vi "Initialisation Spectro.vi"(8 "error in (no error)":errorcluster caption="entrée d'erreur (pas d'erreur)", 10 "Connecter?":bool, 11 "UI SA en entrée":refnum<class "UI SmarAct.lvclass">) -> (0 "error out":errorcluster caption="sortie d'erreur", 1 "Serial Number":string, 2 "Spectrometer Name":string, 3 "UI SA en sortie":refnum<class "UI SmarAct.lvclass">, 4 "Spectro Connecté?":bool)   [LabVIEW 2024, in "UI SmarAct.lvclass"]
uses:
  UI SmarAct.lvclass
  UI SmarAct.lvclass/UI SmarAct.ctl
  d47b7c42-ba51-4529-b271-ce5c7830c4e4.vi
  <vilib>/Utility/error.llb/Error Cluster From Error Code.vi
  <vilib>/ErrorRing/Error Ring.xnode
  Spectro Acquisition/Spectro Acquisition.lvclass
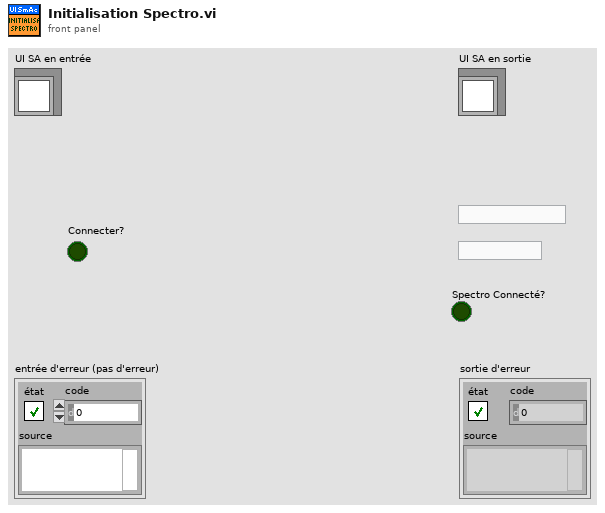
[diagram p1: front panel]
types:
  T1 = enum8{"Enabled", "Disabled", "Disabled and Grayed Out"}
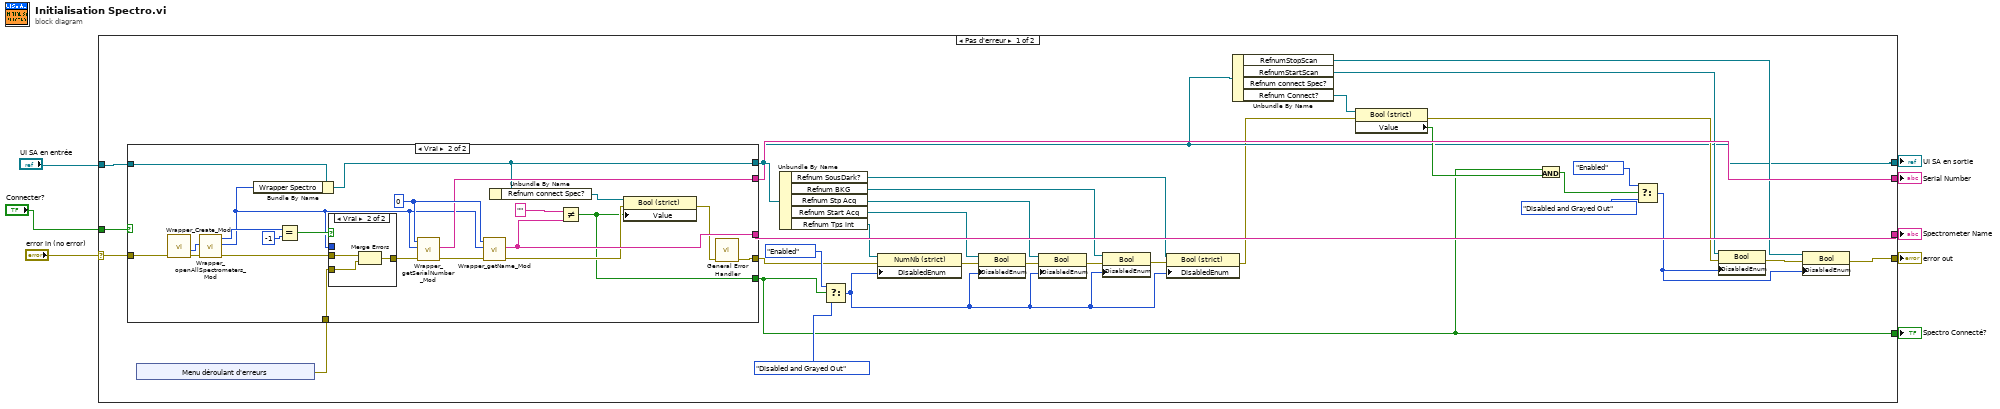
[diagram p0: block diagram]
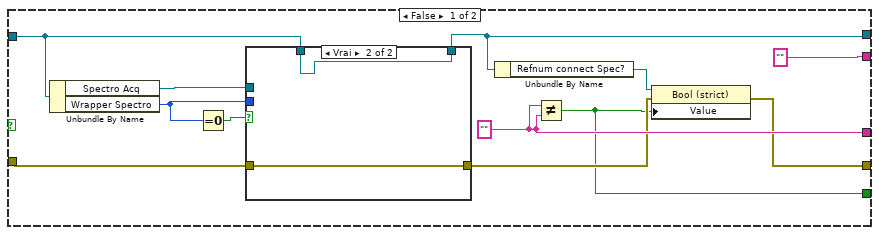
[diagram p2: hidden frame]
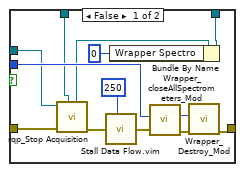
[diagram p3: hidden frame]
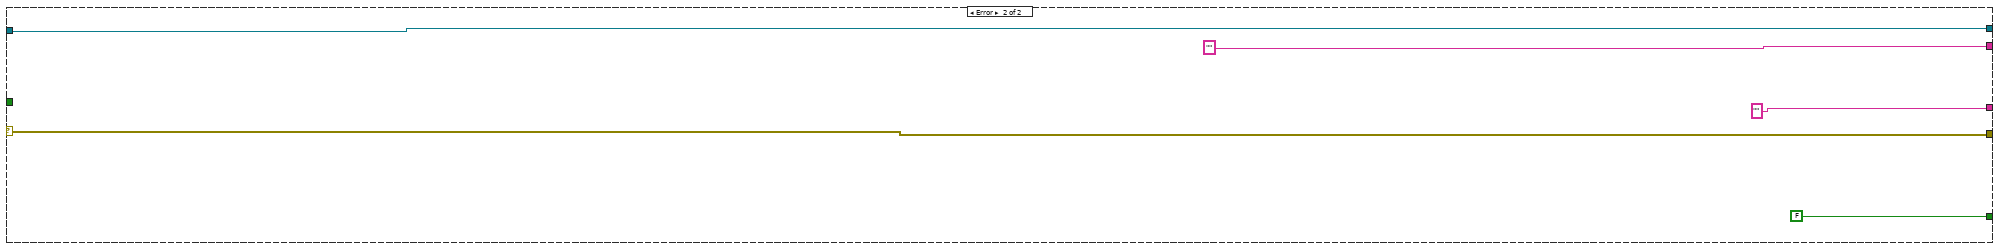
[diagram p5: hidden frame]
diagram:
  n1 = case shown="Pas d'erreur" "error in (no error)" {
    selector: "error in (no error)" -> [w38 w104]
    tunnel: [w10 w104] -> w7
    tunnel: [w12 w103] -> w5
    tunnel: "UI SA en entrée" -> [w39 w103]
    tunnel: [w41 "" ("Spectrometer Name")] -> w4
    tunnel: [w40 "" ("Serial Number")] -> w3
    tunnel: "Connecter?" -> [w36 _]
    tunnel: [w9 FALSE] -> w1
    frame No Error {
      n2 = xnode "Menu déroulant d'erreurs"() -> ("sortie d'erreur"=w37:errorcluster)
      n3 = case shown="Vrai" w36 {
        tunnel: [w48 w77] -> w41
        tunnel: ["" ("Serial Number") w89] -> w40
        tunnel: [w43 w75] -> w12
        tunnel: [w46 w80] -> w24
        tunnel: w39 -> [w44 w79]
        tunnel: w38 -> [w51 w78]
        tunnel: w37 -> [_ w70]
        tunnel: [w45 w71] -> w9
        frame False {
          w48 = "" ("Spectrometer Name")
          n4 = Unbundle By Name(w44) -> ("Spectro Acq"=w42:refnum<class "Spectro Acquisition.lvclass">, "Wrapper Spectro"=w50:u32)
          n5 = Equal To 0?(x=w50) -> (x = 0?=w52:bool)
          n6 = case shown="Vrai" w52 {
            tunnel: [w64 w68] -> w47
            tunnel: w51 -> [w62 w68]
            tunnel: w50 -> [w63 _]
            tunnel: w44 -> [w59 w67]
            tunnel: [w55 w67] -> w43
            tunnel: w42 -> [w57 _]
            frame False {
              n7 = call "rqp_Stop Acquisition.vi"("Caller in"=w59, "error in"=w62, "Spectro Acquisition in"=w57) -> ("error out"=w61:errorcluster, "dup Caller out"=w58:refnum<class "UI SmarAct.lvclass">)  [unwired: 6 in, 1 out]
              n8 = call "Stall Data Flow.vim"("value in"=w61, "milliseconds to wait"=u32 250) -> ("value out"=w60:errorcluster)  [unwired: 1 out]
              n9 = Bundle By Name(cluster=w58, "Wrapper Spectro"=u32 0) -> (w55:refnum<class "UI SmarAct.lvclass">)
              n10 = call "Wrapper_closeAllSpectrometers_Mod.vi"("error in (no error)"=w60, "Wrapper In"=w63) -> ("error out"=w66:errorcluster, "Wrapper Out"=w65:u32)  [unwired: 8 in]
              n11 = call "Wrapper_Destroy_Mod.vi"("error in (no error)"=w66, "Wrapper"=w65) -> ("error out"=w64:errorcluster)  [unwired: 9 in]
            }
            frame True {
            }
          }
          n12 = Unbundle By Name(w43) -> ("Refnum connect Spec?"=w49:refnum<vi>)
          n13 = Not Equal?(x=w48, y=w48) -> (x != y?=w45:bool)
          n14 = property class="Bool (strict)"(reference=w49, error in=w47, "Value"=w45) -> (error out=w46:errorcluster)  [unwired: 1 out]
        }
        frame True {
          w90 = 0 ("Index")
          n15 = call "Wrapper_Create_Mod.vi"("error in (no error)"=w78) -> ("error out"=w85:errorcluster, "Wrapper"=w86:u32)  [unwired: 9 in]
          n16 = call "Wrapper_openAllSpectrometers_Mod.vi"("error in (no error)"=w85, "Wrapper In"=w86) -> ("error out"=w84:errorcluster, "Wrapper Out"=w81:u32, "Number of Spectrometers"=w88:i32)  [unwired: 7 in]
          n17 = Bundle By Name(cluster=w79, "Wrapper Spectro"=w81) -> (w75:refnum<class "UI SmarAct.lvclass">)
          n18 = Equal?(x=w88, y=-1) -> (x = y?=w82:bool)
          n19 = case shown="Vrai" w82 {
            tunnel: w84 -> [w91 w94]
            tunnel: [w91 w93] -> w83
            tunnel: w81 -> [_ _]
            tunnel: w70 -> [_ w92]
            frame False {
            }
            frame True {
              n20 = Merge Errors(w94, w92) -> (w93:errorcluster)
            }
          }
          n21 = call "Wrapper_getSerialNumber_Mod.vi"("error in (no error)"=w83, "Wrapper"=w81, "Index"=w90) -> ("error out"=w69:errorcluster, "Serial Number"=w89:string)  [unwired: 7 in]
          n22 = call "Wrapper_getName_Mod.vi"("error in (no error)"=w69, "Wrapper"=w81, "Index"=w90) -> ("error out"=w73:errorcluster, "Spectrometer Name"=w77:string)  [unwired: 7 in]
          n23 = Unbundle By Name(w75) -> ("Refnum connect Spec?"=w74:refnum<vi>)
          n24 = Not Equal?(x="", y=w77) -> (x != y?=w71:bool)
          n25 = property class="Bool (strict)"(reference=w74, error in=w73, "Value"=w71) -> (error out=w72:errorcluster)  [unwired: 1 out]
          n26 = call <vilib>:"General Error Handler.vi"("error in (no error)"=w72) -> ("error out"=w80:errorcluster)  [unwired: 10 in, 4 out]
        }
      }
      n27 = Unbundle By Name(w12) -> ("Refnum SousDark?"=w26:refnum<vi>, "Refnum BKG"=w27:refnum<vi>, "Refnum Stp Acq"=w28:refnum<vi>, "Refnum Start Acq"=w31:refnum<vi>, "Refnum Tps int"=w35:refnum<vi>)
      n28 = Select(t=T1."Enabled" ("Désactivée"), s=w9, f=T1."Disabled and Grayed Out" ("Désactivée")) -> (s? t:f=w23:T1)
      n29 = property class="NumNb (strict)"(reference=w35, error in=w24, "DisabledEnum"=w23) -> (error out=w32:errorcluster)  [unwired: 1 out]
      n30 = property class="Bool"(reference=w31, error in=w32, "DisabledEnum"=w23) -> (error out=w30:errorcluster)  [unwired: 1 out]
      n31 = property class="Bool"(reference=w28, error in=w30, "DisabledEnum"=w23) -> (error out=w29:errorcluster)  [unwired: 1 out]
      n32 = property class="Bool"(reference=w27, error in=w29, "DisabledEnum"=w23) -> (error out=w25:errorcluster)  [unwired: 1 out]
      n33 = property class="Bool (strict)"(reference=w26, error in=w25, "DisabledEnum"=w23) -> (error out=w11:errorcluster)  [unwired: 1 out]
      n34 = Unbundle By Name(w12) -> ("RefnumStopScan"=w15:refnum<vi>, "RefnumStartScan"=w16:refnum<vi>, "Refnum Connect?"=w22:refnum<vi>)  [unwired: 1 out]
      n35 = property class="Bool (strict)"(reference=w22, error in=w11) -> (error out=w21:errorcluster, "Value"=w20:bool)  [unwired: 1 out]
      n36 = And(x=w9, y=w20) -> (x .and. y?=w17:bool)
      n37 = Select(t=T1."Enabled" ("Désactivée"), s=w17, f=T1."Disabled and Grayed Out" ("Désactivée")) -> (s? t:f=w14:T1)
      n38 = property class="Bool"(reference=w16, error in=w21, "DisabledEnum"=w14) -> (error out=w13:errorcluster)  [unwired: 1 out]
      n39 = property class="Bool"(reference=w15, error in=w13, "DisabledEnum"=w14) -> (error out=w10:errorcluster)  [unwired: 1 out]
    }
    frame Error {
    }
  }
  "error out" <- w7
  "UI SA en sortie" <- w5
  "Spectrometer Name" <- w4
  "Serial Number" <- w3
  "Spectro Connecté?" <- w1
